vi "ExcelInertRows.vi"(8 "error in (no error)":errorcluster, 9 "start (0, 0)":cluster{"row":i32, "column":i32}, 10 "Numeric":i32, 11 "report in":refnum<class "NI_report.lvclass">) -> (0 "error out":errorcluster, 3 "report out":refnum<class "NI_report.lvclass">)   [LabVIEW 2012]
uses:
  <vilib>/Utility/NIReport.llb/NI_report.lvclass
  <vilib>/Utility/NIReport.llb/Excel/NI_Excel.lvclass
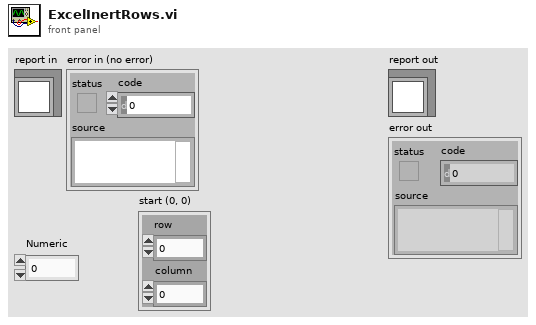
[diagram p1: front panel]
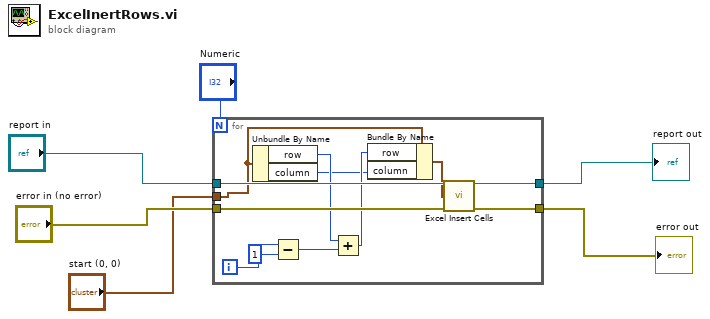
[diagram p0: block diagram]
diagram:
  n1 = for {
    N: "Numeric" -> [_]
    tunnel: "report in" -> [w18]
    tunnel: "error in (no error)" -> [w17]
    tunnel: [w16] -> w4
    tunnel: [w15] -> w3
    tunnel: "start (0, 0)" -> [w10]
    i -> [w14]
    n2 = Unbundle By Name(w10) -> ("row"=w11:i32, "column"=w7:i32)
    n3 = Subtract(x=w14, y=1) -> (x-y=w12:i32)
    n4 = Add(x=w11, y=w12) -> (x+y=w8:i32)
    n5 = Bundle By Name(cluster=w10, "row"=w8, "column"=w7) -> (w9:cluster{"row":i32, "column":i32})
    n6 = call <vilib>:"Excel Insert Cells.vi"("report in"=w18, "start (0, 0)"=w9, "error in (no error)"=w17) -> ("report out"=w16:refnum<class "NI_report.lvclass">, "error out"=w15:errorcluster)  [unwired: 11 in]
  }
  "report out" <- w4
  "error out" <- w3
